vi "Toggle.vi"(7 "Control":bool=TRUE, 10 "Input":bool) -> (2 "Output":bool)   [LabVIEW 2016]
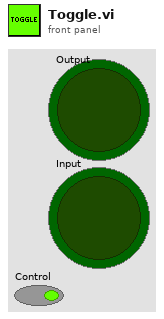
[diagram p1: front panel]
types:
  T1 = typedef "WPI_DriverStationRobotMode2.ctl" = enum16{"Autonomous Disabled", "Autonomous Enabled", "Teleop Disabled", "Teleop Enabled", "Disconnected", "Finish", "Test Disabled", "Test Enabled", "Emergency Stopped"}
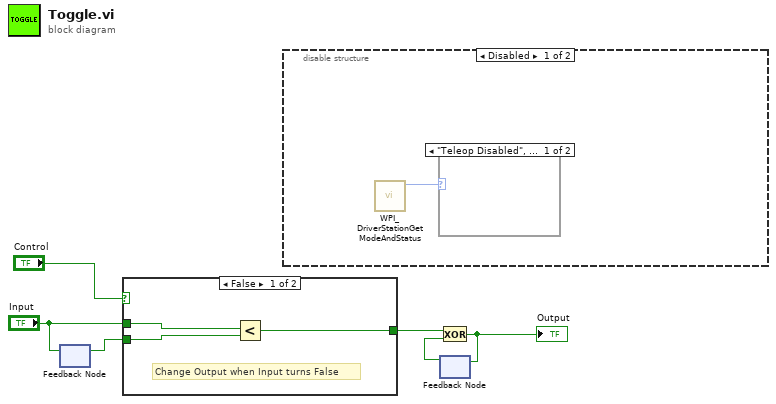
[diagram p0: block diagram]
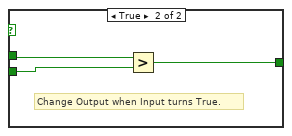
[diagram p4: hidden frame]
diagram:
  n1 = feedback #1() -> (w4:bool)  [unwired: 1 in]
  n2 = feedback-in #1("Input") -> ()
  n3 = case shown="False" "Control" {
    tunnel: [w9 w12] -> w5
    tunnel: w4 -> [w8 w10]
    tunnel: "Input" -> [w7 w11]
    frame False {
      # "Change Output when Input turns False"
      n4 = Less?(x=w7, y=w8) -> (x < y?=w9:bool)
    }
    frame True {
      # "Change Output when Input turns True."
      n5 = Greater?(x=w11, y=w10) -> (0:w12:bool)
    }
  }
  n6 = disable-structure shown="Disabled" {
    frame Disabled {
      n7 = call <vilib>:"WPI_DriverStationGetModeAndStatus.vi"() -> ("Robot Mode"=w13:T1)  [unwired: 10 in, 1 out]
      n8 = case shown="\"Teleop Disabled\", Default" w13 {
        frame "Teleop Disabled", Default {
        }
        frame "Teleop Enabled" {
        }
      }
    }
    frame Enabled {
    }
  }
  n9 = feedback #2() -> (w6:bool)  [unwired: 1 in]
  n10 = Exclusive Or(1:w6, 2:w5) -> (0:w1:bool)
  "Output" <- w1
  n11 = feedback-in #2(w1) -> ()
